vi "Get_string_subset.vi"(2 "String Name":string, 3 "Show Dialog?":bool, 4 "String to split":string, 5 "File Label":string) -> (0 "Status":enum16{"Char in string", "Char not in string"}(ring), 1 "Output string":string)   [LabVIEW 2020]
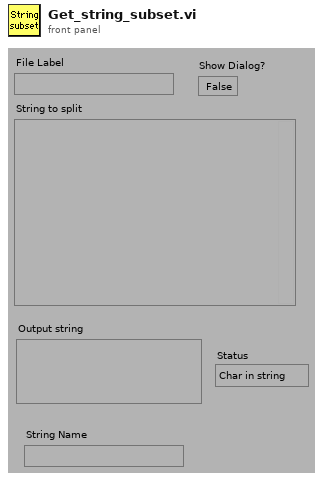
[diagram p1: front panel]
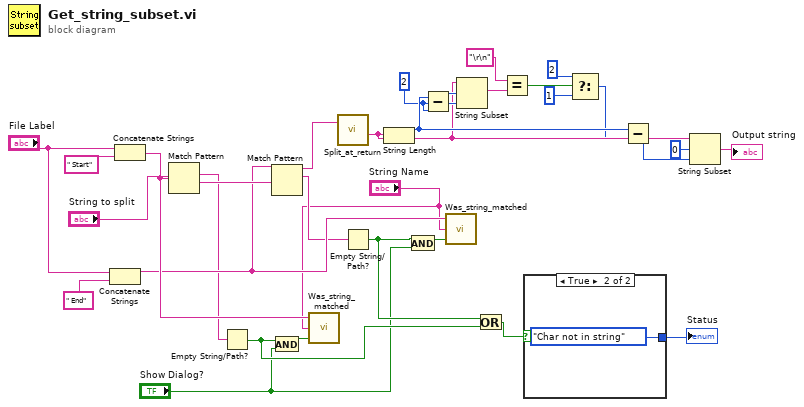
[diagram p0: block diagram]
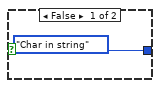
[diagram p2: hidden frame]
diagram:
  w6 = 2 ("length")
  n1 = Concatenate Strings("File Label", " End") -> (w25:string)
  n2 = Concatenate Strings("File Label", " Start") -> (w26:string)
  n3 = Match Pattern(string="String to split", regular expression=w26) -> (match substring=w23:string, after substring=w27:string)  [unwired: 3 out]
  n4 = Empty String/Path?(string/path=w23) -> (empty?=w13:bool)
  n5 = Match Pattern(string=w27, regular expression=w25) -> (before substring=w8:string, match substring=w24:string)  [unwired: 3 out]
  n6 = And(x=w13, y="Show Dialog?") -> (x .and. y?=w12:bool)
  n7 = call "Was_string_matched.vi"("Match Error"=w12, "String Name"="String Name", "Variable name"=w26) -> ()
  n8 = call "Split_at_return.vi"("String"=w8) -> ("after substring"=w4:string)  [unwired: 1 in, 3 out]
  n9 = Empty String/Path?(string/path=w24) -> (empty?=w11:bool)
  n10 = String Length(string=w4) -> (length=w7:i32)
  n11 = And(x=w11, y="Show Dialog?") -> (x .and. y?=w10:bool)
  n12 = Subtract(x=w7, y=w6) -> (x-y=w5:i32)
  n13 = call "Was_string_matched.vi"("Match Error"=w10, "String Name"="String Name", "Variable name"=w25) -> ()
  n14 = String Subset(string=w4, offset (0)=w5, length (rest)=w6) -> (substring=w20:string)
  n15 = Or(x=w11, y=w13) -> (x .or. y?=w14:bool)
  n16 = Equal?(x="\r\n", y=w20) -> (x = y?=w18:bool)
  n17 = case shown="True" w14 {
    tunnel: [enum16{"Char in string", "Char not in string"}."Char in string" enum16{"Char in string", "Char not in string"}."Char not in string"] -> w15
    frame False {
    }
    frame True {
    }
  }
  "Status" <- w15
  n18 = Select(t=2 ("y"), s=w18, f=1) -> (s? t:f=w2:i32)
  n19 = Subtract(x=w7, y=w2) -> (x-y=w22:i32)
  n20 = String Subset(string=w4, offset (0)=0, length (rest)=w22) -> (substring=→"Output string":string)
